vi "SPECTRUM Get Trace.vi"(7 "outTracePoints":i32, 8 "error in (no error)":errorcluster, 9 "traceData":sgl[](array[numeric]), 10 "maxTracePoints":i32, 11 "trace":u32(ring) items=["SpectrumTrace1", "SpectrumTrace2", "SpectrumTrace3"]) -> (0 "error out":errorcluster, 1 "traceData out":sgl[](array[numeric]), 3 "function return":u32(ring), 5 "outTracePoints out":i32)   [LabVIEW 2016, in "RSA_API.lvlib"]
doc: "RSA_API_DLL ReturnStatus SPECTRUM_GetTrace(SpectrumTraces trace, int maxTracePoints, float *traceData, int *outTracePoints);"
uses:
  <userlib>/RSA_API/RSA_API.lvlib
  Tektronix/RSA_API/lib/x86/RSA_API.dll
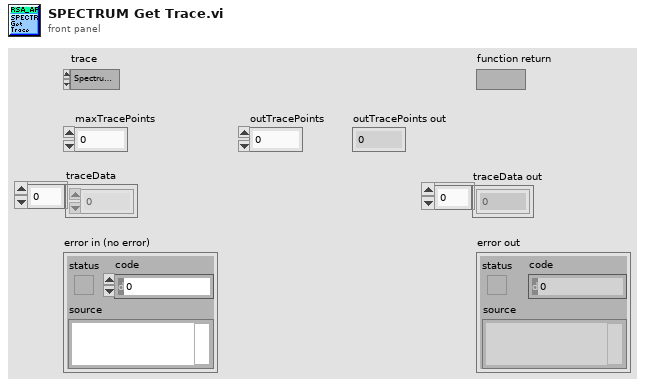
[diagram p1: front panel]
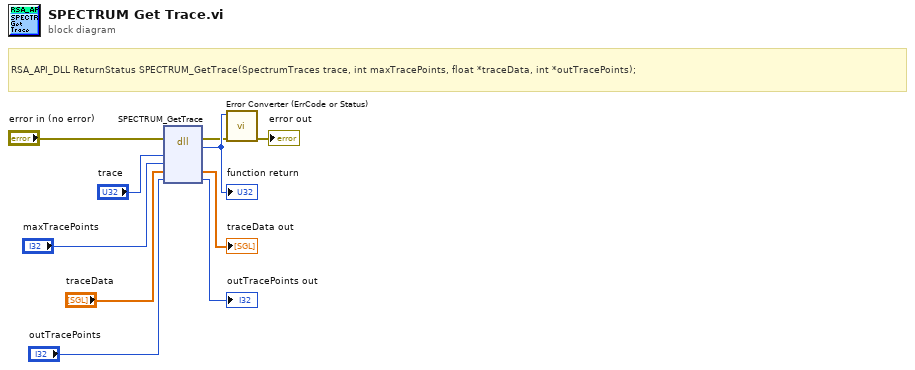
[diagram p0: block diagram]
diagram:
  # "RSA_API_DLL ReturnStatus SPECTRUM_GetTrace(SpectrumTraces trace, int maxTracePoints, float *traceData, int *outTracePoints);"
  n1 = dll-call lib="C:/Tektronix/RSA_API/lib/x86/RSA_API.dll" fn="SPECTRUM_GetTrace"(error in="error in (no error)", "trace"="trace", "maxTracePoints"="maxTracePoints", "traceData"="traceData", "outTracePoints"="outTracePoints") -> (error out=w2:errorcluster, "return type"=w10:u32, "traceData"=→"traceData out":sgl[], "outTracePoints"=→"outTracePoints out":i32)  [unwired: 4 in, 1 out]
  "function return" <- w10
  n2 = call <userlib>:"Error Converter (ErrCode or Status).vi"("error in (no error)"=w2, "error code"=w10) -> ("error out"=→"error out":errorcluster)  [unwired: 9 in]
